vi "Arrange VIWin - Resize BD.vi"(0 "VI in":refnum<vi>, 1 "BD canvas margin":i16, 5 "Window INI tokens":T4, 11 "error in":errorcluster) -> (15 "error out":errorcluster)   [LabVIEW 2012, in "Arrange VI Window.lvlib"]
uses:
  Arrange VI Window.lvlib
  <vilib>/Utility/miscctls.llb/LVRectTypeDef.ctl
  Arrange VIWin - Min Window Dimensions.ctl
  Arrange VIWin - Window Gaps.ctl
  <vilib>/Utility/miscctls.llb/LVPointTypeDef.ctl
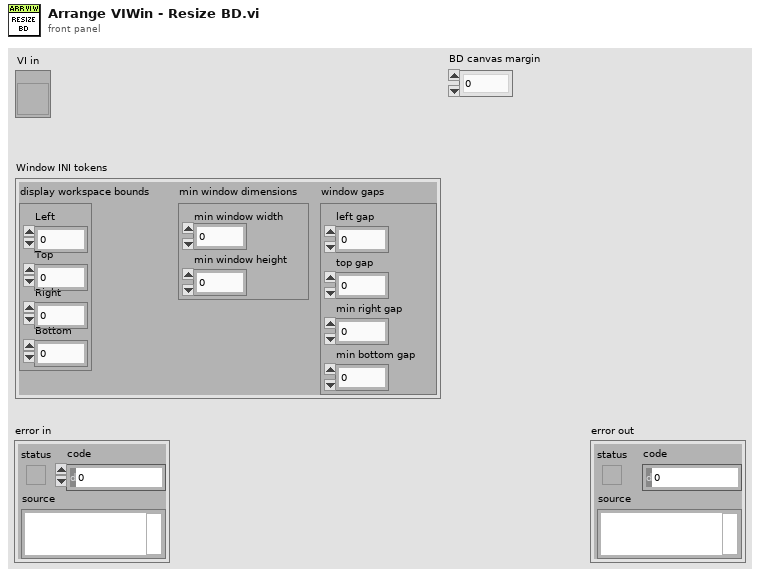
[diagram p1: front panel]
types:
  T1 = typedef "LVRectTypeDef.ctl" = cluster{"Left":i16, "Top":i16, "Right":i16, "Bottom":i16}
  T2 = typedef "Arrange VI Window.lvlib/Arrange VIWin - Min Window Dimensions.ctl" = cluster{"min window width":i16, "min window height":i16}
  T3 = typedef "Arrange VI Window.lvlib/Arrange VIWin - Window Gaps.ctl" = cluster{"left gap":i16, "top gap":i16, "min right gap":i16, "min bottom gap":i16}
  T4 = cluster{"display workspace bounds":T1, "min window dimensions":T2, "window gaps":T3}
  T5 = typedef "LVPointTypeDef.ctl" = cluster{"Horizontal":i16, "Vertical":i16}
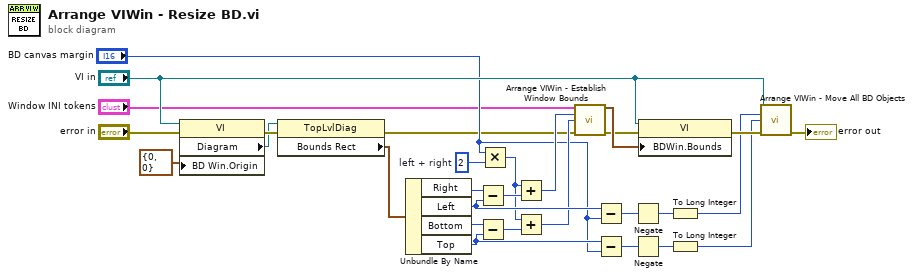
[diagram p0: block diagram]
diagram:
  w9 = i16 2  # left + right
  n1 = property on="Property Node" class="VI"(reference="VI in", error in="error in", "BD Win.Origin"=T5 {"Horizontal"=0, "Vertical"=0} ("Block Diagram Window:Origin")) -> (error out=w29:errorcluster, "Diagram"=w11:refnum<vi>)  [unwired: 1 out]
  n2 = property on="Property Node" class="TopLvlDiag"(reference=w11, error in=w29) -> (error out=w2:errorcluster, "Bounds Rect"=w16:T1)  [unwired: 1 out]
  n3 = Unbundle By Name(w16) -> ("Right"=w26:i16, "Left"=w19:i16, "Bottom"=w27:i16, "Top"=w18:i16)
  n4 = Subtract(x=w26, y=w19) -> (x-y=w23:i16)
  n5 = Subtract(x=w27, y=w18) -> (x-y=w22:i16)
  n6 = Multiply(x="BD canvas margin", y=w9) -> (x*y=w6:i16)
  n7 = Add(x=w6, y=w23) -> (x+y=w8:i16)
  n8 = Add(x=w6, y=w22) -> (x+y=w7:i16)
  n9 = call "Arrange VIWin - Establish Window Bounds.vi"("Window INI tokens"="Window INI tokens", "content rectangle width"=w8, "content rectangle height"=w7, "error in"=w2) -> ("window bounds"=w28:T1, "error out"=w24:errorcluster)  [unwired: 10 in]
  n10 = Subtract(x=w19, y="BD canvas margin") -> (x-y=w5:i16)
  n11 = Subtract(x=w18, y="BD canvas margin") -> (x-y=w4:i16)
  n12 = Negate(x=w5) -> (-x=w15:i16)
  n13 = Negate(x=w4) -> (-x=w14:i16)
  n14 = property on="Property Node" class="VI"(reference="VI in", error in=w24, "BDWin.Bounds"=w28) -> (error out=w20:errorcluster)  [unwired: 1 out]
  n15 = To Long Integer(number=w15) -> (32bit integer=w13:i32)
  n16 = To Long Integer(number=w14) -> (32bit integer=w12:i32)
  n17 = call "Arrange VIWin - Move All BD Objects.vi"("VI in"="VI in", "x delta"=w13, "y delta"=w12, "error in"=w20) -> ("error out"=→"error out":errorcluster)  [unwired: 11 in]
